vi "3D Height Map.vi"(9 "scan data":dbl[][](array[numeric])) -> (1 "3D Picture":refnum<vi>(3d-picture))   [LabVIEW 2023]
uses:
  <vilib>/picture/3D Picture Control/NI_3D Picture Control.lvlib
  <vilib>/picture/3D Picture Control/Object/Create Object (name).vi
  <vilib>/Utility/miscctls.llb/LV3DPointTypeDef.ctl
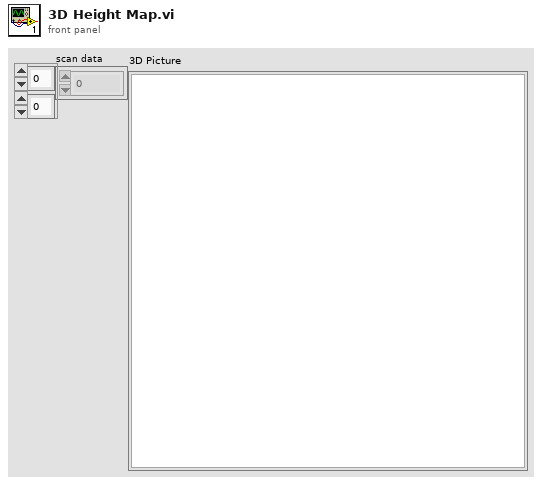
[diagram p1: front panel]
types:
  T1 = typedef "LV3DPointTypeDef.ctl" = cluster{"X":sgl, "Y":sgl, "Z":sgl}
  T2 = cluster{"Red":sgl, "Green":sgl, "Blue":sgl, "Alpha":sgl}
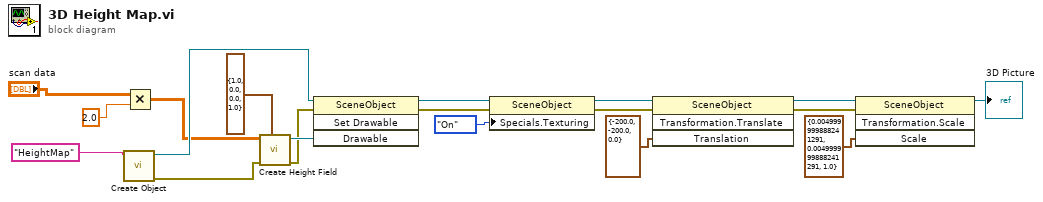
[diagram p0: block diagram]
diagram:
  n1 = call-poly <vilib>:"Create Object.vi"("Name"="HeightMap") -> ("error out"=w19:errorcluster, "Scene:New Object"=w17:refnum<vi>)  [unwired: 9 in]
  n2 = Multiply(x="scan data", y=2.0) -> (x*y=w11:dbl[][])
  n3 = call <vilib>:"Create Height Field.vi"("Color"=T2 {"Red"=1.0, "Green"=0.0, "Blue"=0.0, "Alpha"=1.0}, "error in (no error)"=w19, "Data"=w11) -> ("error out"=w4:errorcluster, "New Height Field Refnum"=w16:refnum<vi>)  [unwired: 7 in]
  n4 = invoke class="SceneObject" method="Set Drawable"(reference=w17, error in=w4, "Drawable"=w16) -> (reference out=w15:refnum<vi>, error out=w14:errorcluster)  [unwired: 1 in, 2 out]
  n5 = property class="SceneObject"(reference=w15, error in=w14, "Specials.Texturing"=enum16{"Inherit Value", "Off", "On"}."On" ("Specials:Texturing")) -> (reference out=w6:refnum<vi>, error out=w5:errorcluster)
  n6 = invoke class="SceneObject" method="Transformation.Translate"(reference=w6, error in=w5, "Translation"=T1 {"X"=-200.0, "Y"=-200.0, "Z"=0.0} ("Axis")) -> (reference out=w10:refnum<vi>, error out=w9:errorcluster)  [unwired: 1 in, 2 out]
  n7 = invoke class="SceneObject" method="Transformation.Scale"(reference=w10, error in=w9, "Scale"=T1 {"X"=0.005, "Y"=0.005, "Z"=1.0}) -> (reference out=→"3D Picture":refnum<vi>)  [unwired: 1 in, 3 out]
